vi "fil ter matrix.vi"(7 "matrix":dbl[](array[numeric])=array[4097 elements], 8 "error in (no error)":errorcluster, 9 "multiplication/ substitution":i16(ring) items=["subst", "mult"], 10 "intensity / phase":i16(ring) items=["int", "pha"], 11 "field":T1) -> (0 "error out":errorcluster, 3 "field out":T1, 5 "matrix out":dbl[](array[numeric]))   [LabVIEW 2012, in "Lightpipes.lvlib"]
doc: "__declspec(dllexport) void fil_ter_matrix(FIELD* field, const char* c1, const char* c2, double matrix[]);"
uses:
  LightPipes.lvlib
  Lightpipes.dll
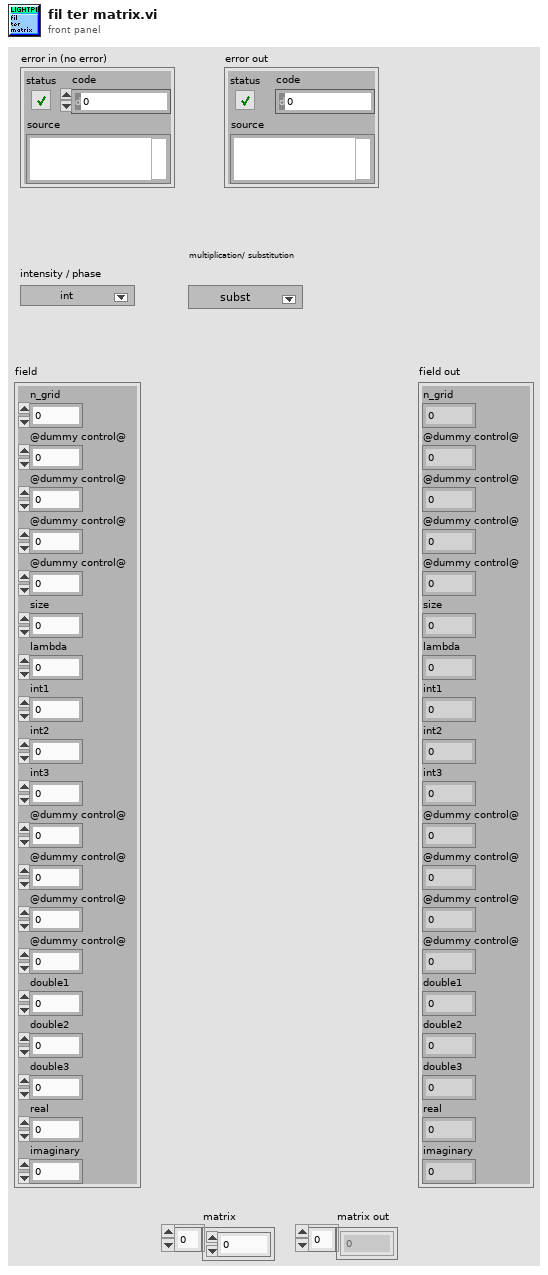
[diagram p1: front panel]
types:
  T1 = cluster{"n_grid":i32, "@dummy control@":i8, "@dummy control@":i8, "@dummy control@":i8, "@dummy control@":i8, "size":dbl, "lambda":dbl, "int1":i32, "int2":i32, "int3":i32, "@dummy control@":i8, "@dummy control@":i8, "@dummy control@":i8, "@dummy control@":i8, "double1":dbl, "double2":dbl, "double3":dbl, "real":u32, "imaginary":u32}
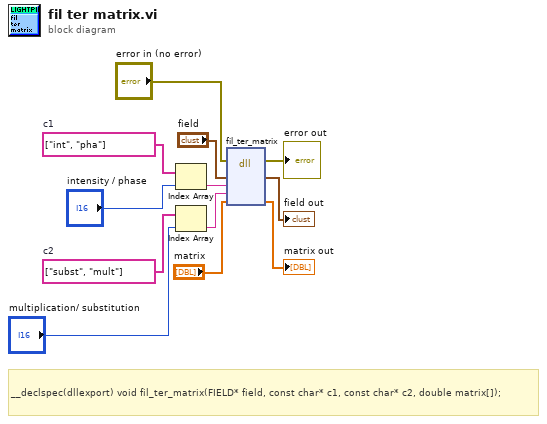
[diagram p0: block diagram]
diagram:
  w6 = string[] ["int", "pha"]  # c1
  w8 = string[] ["subst", "mult"]  # c2
  # "__declspec(dllexport) void fil_ter_matrix(FIELD* field, const char* c1, const char* c2, double matrix[]);"
  n1 = Index Array(array=w6, index="intensity / phase") -> (element=w4:string)
  n2 = Index Array(array=w8, index="multiplication/ substitution") -> (element=w3:string)
  n3 = dll-call lib="C:/Users/Tri/Documents/Gerchberg/Lightpipes.*" fn="fil_ter_matrix"(error in="error in (no error)", "field"="field", "c1"=w4, "c2"=w3, "matrix"="matrix") -> (error out=→"error out":errorcluster, "field"=→"field out":T1, "matrix"=→"matrix out":dbl[])  [unwired: 5 in, 1 out]
